vi "coffemachine.vi"() -> ()   [LabVIEW 2023]
uses:
  CoffeeStateMachineControl.ctl
panel:
  out "SUgar":dbl
  out "Tank":dbl(slide) scale=0.0..100.0
  in  "Exit":bool
  in  "Choco":bool
  in  "Cappucino":bool
  in  "Espresso":bool
  out "Numeric":i32
  out "Enum":T1
  # "1.Creare Enum pentru stari\n1a. Enum --> Type Definition\n2.Implementare Finite State Machine\n2a. While Loop\n2b.Shift Register - tranzitii\n2c.Cases - starile\n2ci. Creare stari in case\n2d.Deal with exit"
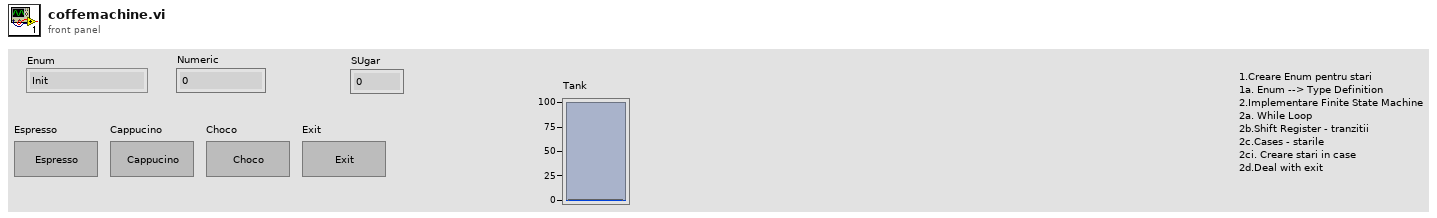
[diagram p1: front panel]
types:
  T1 = typedef "CoffeeStateMachineControl.ctl" = enum16{"Init", "Wait", "Espresso", "Cappucino", "Ciocolata", "Sugar", "Lapte Spuma", "Lapte Normal", "Ciocolata Alba", "Delivery", "Exit", "Black Choco"}
  T2 = enum16{"Left Button", "Center Button", "Right Button", "Window Close"}
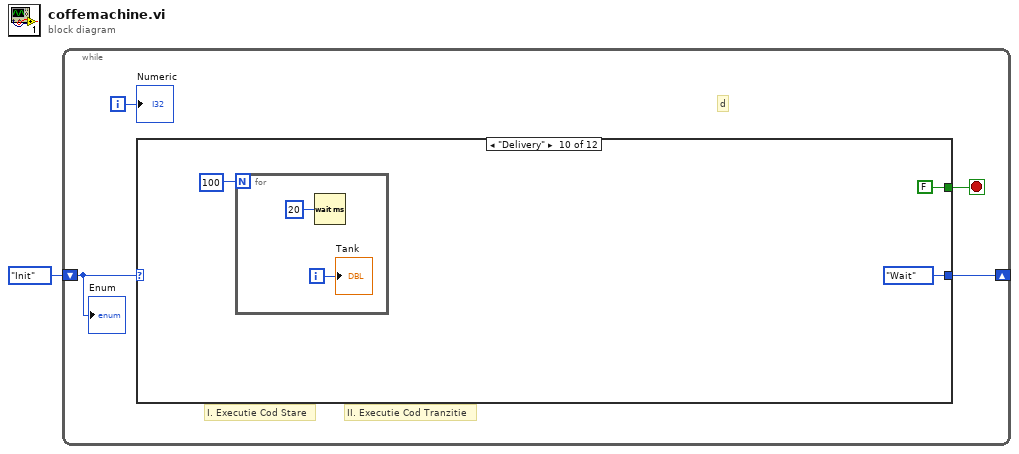
[diagram p0: block diagram]
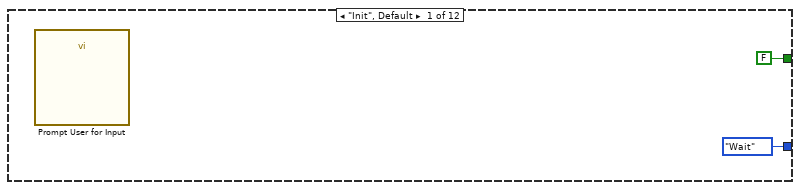
[diagram p2: hidden frame]
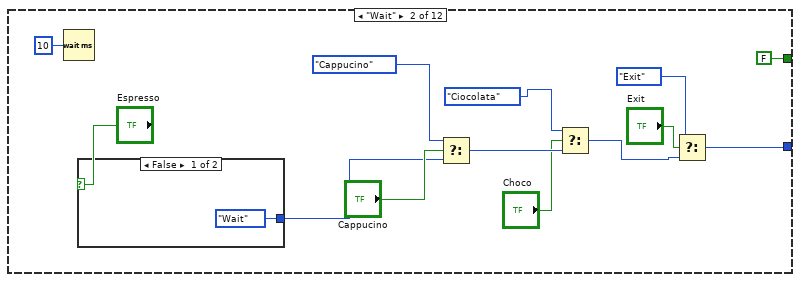
[diagram p3: hidden frame]
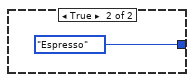
[diagram p4: hidden frame]
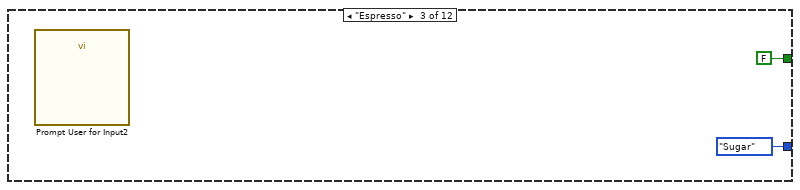
[diagram p5: hidden frame]
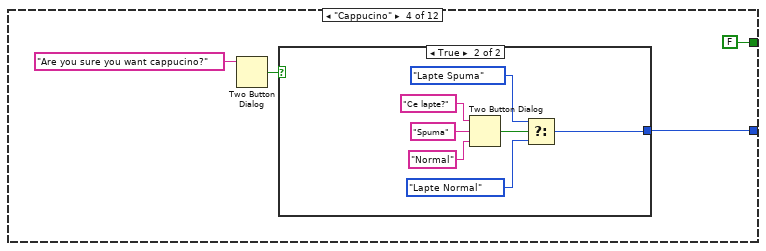
[diagram p6: hidden frame]
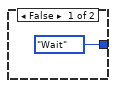
[diagram p7: hidden frame]
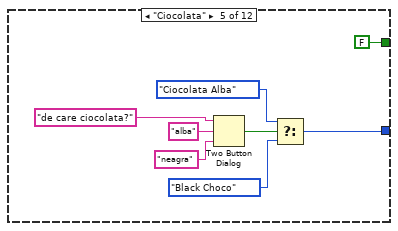
[diagram p8: hidden frame]
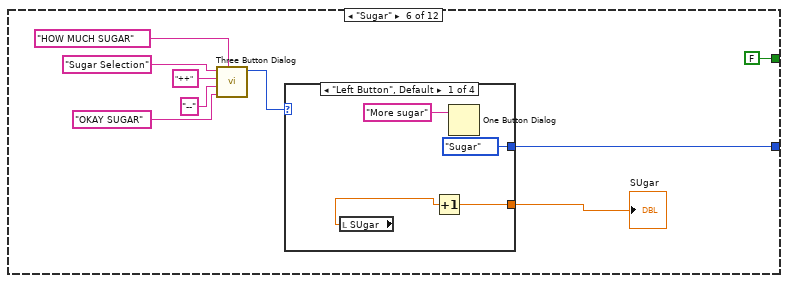
[diagram p9: hidden frame]
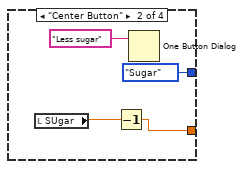
[diagram p10: hidden frame]
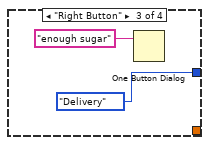
[diagram p11: hidden frame]
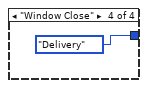
[diagram p12: hidden frame]
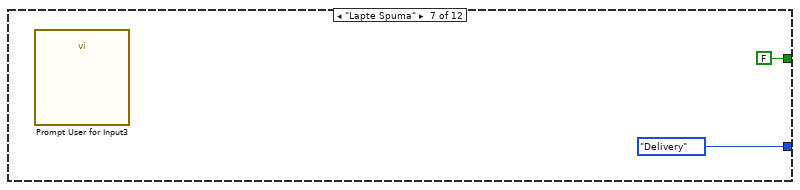
[diagram p13: hidden frame]
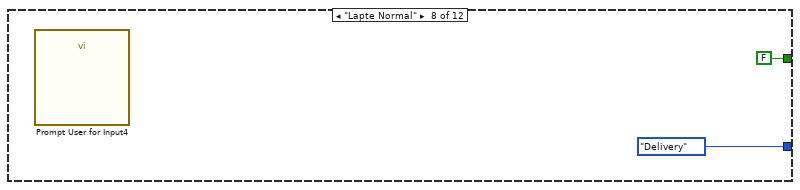
[diagram p14: hidden frame]
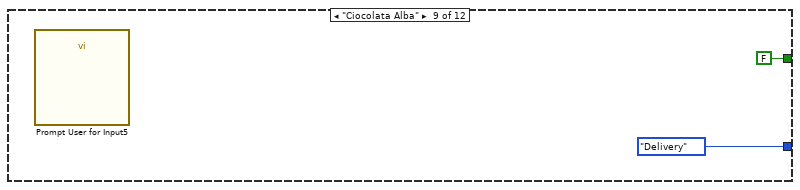
[diagram p15: hidden frame]
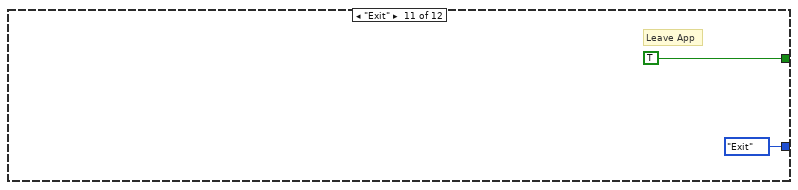
[diagram p16: hidden frame]
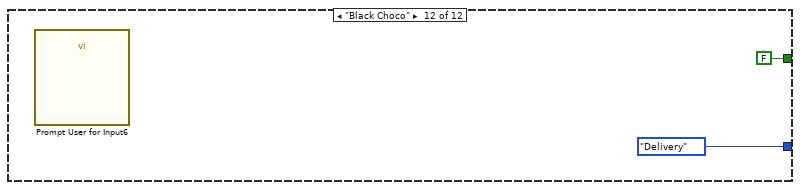
[diagram p17: hidden frame]
diagram:
  n1 = while {
    shift-right: [w3] -> _
    shift-left: CoffeeStateMachineControl."Init" ("Enum") -> [w2]
    i -> [w5]
    stop <- w4 stop-if-true
    # "d"
    # "II. Executie Cod Tranzitie"
    # "I. Executie Cod Stare"
    n2 = case shown="\"Delivery\"" w2 {
      tunnel: [FALSE FALSE FALSE FALSE FALSE FALSE FALSE FALSE FALSE FALSE TRUE FALSE] -> w4
      tunnel: [CoffeeStateMachineControl."Wait" ("Enum") w10 CoffeeStateMachineControl."Sugar" ("Enum") w26 w38 w45 CoffeeStateMachineControl."Delivery" ("Enum") CoffeeStateMachineControl."Delivery" ("Enum") CoffeeStateMachineControl."Delivery" ("Enum") CoffeeStateMachineControl."Wait" ("Enum") CoffeeStateMachineControl."Exit" ("Enum") CoffeeStateMachineControl."Delivery" ("Enum")] -> w3
      frame "Init", Default {
        n3 = call "Prompt User for Input"() -> ()  [unwired: 18 in, 2 out]
      }
      frame "Wait" {
        n4 = Wait (ms)(milliseconds to wait=u32 10) -> ()  [unwired: 1 out]
        n5 = case shown="False" "Espresso" {
          tunnel: [CoffeeStateMachineControl."Wait" ("Enum") CoffeeStateMachineControl."Espresso" ("Enum")] -> w18
          frame False {
          }
          frame True {
          }
        }
        n6 = Select(t=CoffeeStateMachineControl."Cappucino" ("Enum"), s="Cappucino", f=w18) -> (s? t:f=w16:T1)
        n7 = Select(t=CoffeeStateMachineControl."Ciocolata" ("Enum"), s="Choco", f=w16) -> (s? t:f=w12:T1)
        n8 = Select(t=CoffeeStateMachineControl."Exit" ("Enum"), s="Exit", f=w12) -> (s? t:f=w10:T1)
      }
      frame "Espresso" {
        n9 = call "Prompt User for Input2"() -> ()  [unwired: 18 in, 2 out]
      }
      frame "Cappucino" {
        n10 = Two Button Dialog(message="Are you sure you want cappucino?") -> (T button?=w27:bool)  [unwired: 2 in]
        n11 = case shown="True" w27 {
          tunnel: [CoffeeStateMachineControl."Wait" ("Enum") w30] -> w26
          frame False {
          }
          frame True {
            n12 = Two Button Dialog(message="Ce lapte?", 1:"Normal" ("F button name (\"Cancel\")"), 2:"Spuma" ("T button name (\"OK\")")) -> (T button?=w33:bool)
            n13 = Select(t=CoffeeStateMachineControl."Lapte Spuma" ("Enum"), s=w33, f=CoffeeStateMachineControl."Lapte Normal" ("Enum")) -> (s? t:f=w30:T1)
          }
        }
      }
      frame "Ciocolata" {
        n14 = Two Button Dialog(message="de care ciocolata?", 1:"neagra" ("F button name (\"Cancel\")"), 2:"alba" ("T button name (\"OK\")")) -> (T button?=w41:bool)
        n15 = Select(t=CoffeeStateMachineControl."Ciocolata Alba" ("Enum"), s=w41, f=CoffeeStateMachineControl."Black Choco" ("Enum")) -> (s? t:f=w38:T1)
      }
      frame "Sugar" {
        n16 = call <vilib>:"Three Button Dialog.vi"("Window Title (\"\")"="HOW MUCH SUGAR" ("Window Title (\"\")"), "Right Button Text (\"Cancel\")"="OKAY SUGAR" ("Right Button Text (\"Cancel\")"), "Center Button Text (\"No\")"="--" ("Center Button Text (\"No\")"), "Left Button Text (\"Yes\")"="++" ("Left Button Text (\"Yes\")"), "message"="Sugar Selection") -> ("Which Button?"=w48:T2)  [unwired: 6 in]
        n17 = case shown="\"Left Button\", Default" w48 {
          tunnel: [w55 w59 _ _] -> w46
          tunnel: [CoffeeStateMachineControl."Sugar" ("Enum") CoffeeStateMachineControl."Sugar" ("Enum") CoffeeStateMachineControl."Delivery" ("Enum") CoffeeStateMachineControl."Delivery" ("Enum")] -> w45
          frame "Left Button", Default {
            n18 = local read "SUgar"() -> (w56:dbl)
            n19 = Increment(x=w56) -> (x+1=w55:dbl)
            n20 = One Button Dialog(message="More sugar") -> ()  [unwired: 1 in, 1 out]
          }
          frame "Center Button" {
            n21 = local read "SUgar"() -> (w60:dbl)
            n22 = Decrement(x=w60) -> (x-1=w59:dbl)
            n23 = One Button Dialog(message="Less sugar") -> ()  [unwired: 1 in, 1 out]
          }
          frame "Right Button" {
            n24 = One Button Dialog(message="enough sugar") -> ()  [unwired: 1 in, 1 out]
          }
          frame "Window Close" {
          }
        }
        "SUgar" <- w46
      }
      frame "Lapte Spuma" {
        n25 = call "Prompt User for Input3"() -> ()  [unwired: 18 in, 2 out]
      }
      frame "Lapte Normal" {
        n26 = call "Prompt User for Input4"() -> ()  [unwired: 18 in, 2 out]
      }
      frame "Ciocolata Alba" {
        n27 = call "Prompt User for Input5"() -> ()  [unwired: 18 in, 2 out]
      }
      frame "Delivery" {
        n28 = for {
          N: 100 -> [_]
          i -> [w74]
          n29 = Wait (ms)(milliseconds to wait=u32 20) -> ()  [unwired: 1 out]
          "Tank" <- w74
        }
      }
      frame "Exit" {
        # "Leave App"
      }
      frame "Black Choco" {
        n30 = call "Prompt User for Input6"() -> ()  [unwired: 18 in, 2 out]
      }
    }
    "Numeric" <- w5
    "Enum" <- w2
  }
